vi "FTW-Ether-Address-Build.vi"(5 "Path":string, 7 "Message Transport Scheme":T1, 11 "error in":errorcluster) -> (6 "Endpoint Address":string, 15 "error out":errorcluster)   [LabVIEW 2015, in "FTW-Ether.lvclass"]
uses:
  FTW-Ether.lvclass
  FTW-Ether-MessageTransportScheme.ctl
panel:
  # "Inputs"
  # "Outputs"
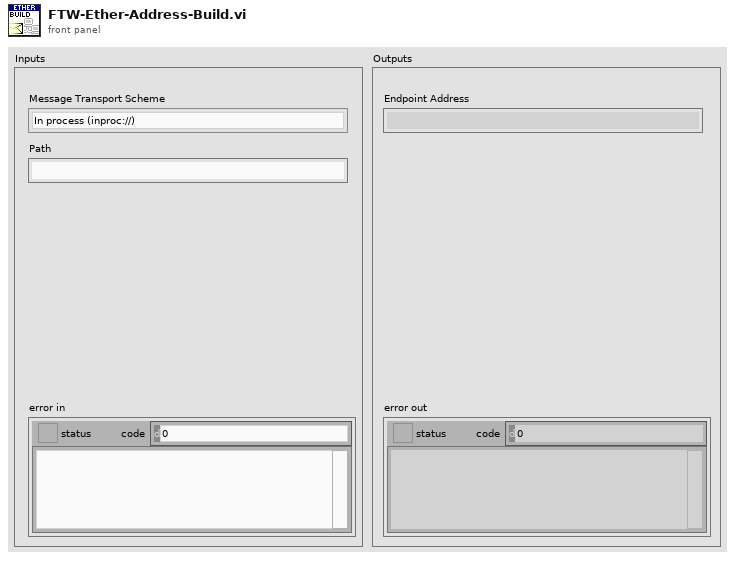
[diagram p1: front panel]
types:
  T1 = typedef "FTW-Ether.lvclass/FTW-Ether-MessageTransportScheme.ctl" = enum16{"In process (inproc://)", "TCP (tcp://)"}
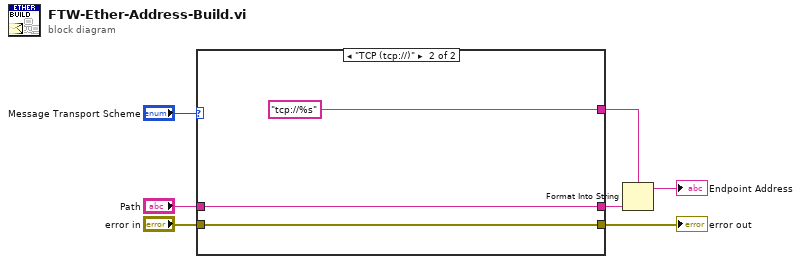
[diagram p0: block diagram]
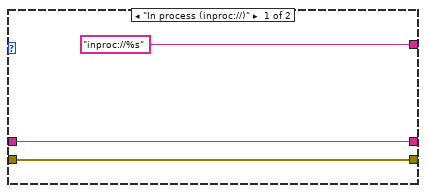
[diagram p2: hidden frame]
diagram:
  n1 = case shown="\"TCP (tcp://)\"" "Message Transport Scheme" {
    tunnel: ["inproc://%s" ("format string") "tcp://%s" ("format string")] -> w6
    tunnel: "Path" -> [w9 w11]
    tunnel: [w9 w11] -> w3
    tunnel: "error in" -> [w8 w12]
    tunnel: [w8 w12] -> w1
    frame "In process (inproc://)" {
    }
    frame "TCP (tcp://)" {
    }
  }
  "error out" <- w1
  n2 = Format Into String(format string=w6, w3) -> (resulting string=→"Endpoint Address":string)  [unwired: 2 in, 1 out]
